vi "NextObject.vi"(8 "error in (no error)":errorcluster, 11 "Iterator":refnum<class "Iterator.lvclass">) -> (0 "error out":errorcluster, 2 "BrowerComponent":refnum<class "BrowerComponent.lvclass">, 3 "Iterator out":refnum<class "Iterator.lvclass">)   [LabVIEW 2015, in "Iterator.lvclass"]
uses:
  Iterator.lvclass
  BrowerComponent/BrowerComponent/BrowerComponent.lvclass
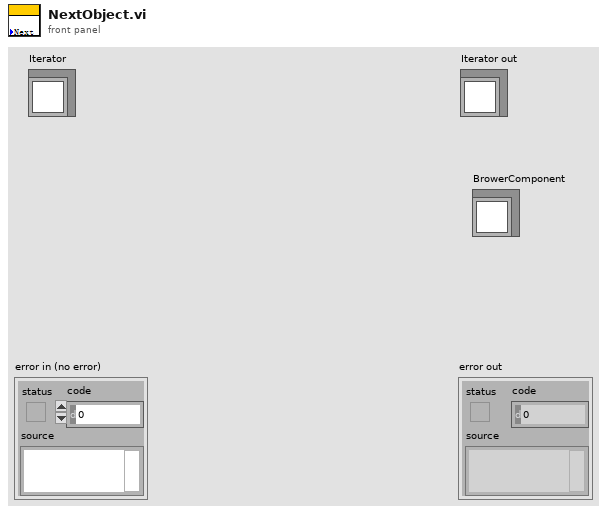
[diagram p1: front panel]
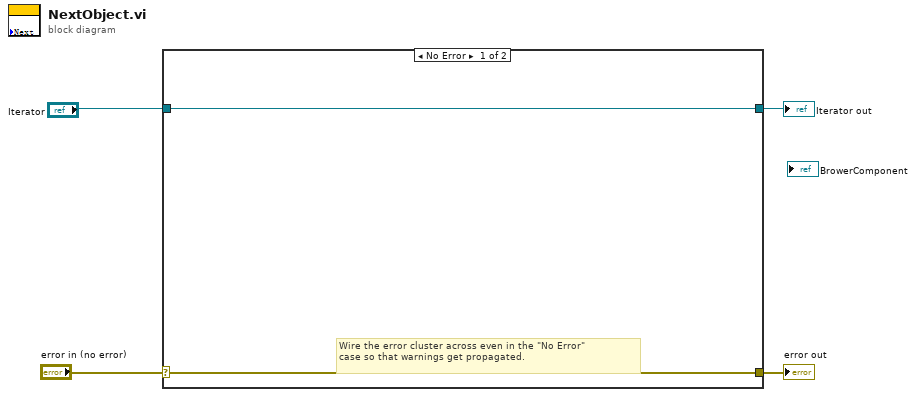
[diagram p0: block diagram]
diagram:
  n1 = case shown="No Error" "error in (no error)" {
    selector: "error in (no error)" -> [w5 w8]
    tunnel: [w5 w8] -> w3
    tunnel: [w6 w7] -> w1
    tunnel: "Iterator" -> [w6 w7]
    frame No Error {
      # "Wire the error cluster across even in the \"No Error\"\ncase so that warnings get propagated."
    }
    frame Error {
    }
  }
  "error out" <- w3
  "Iterator out" <- w1
